vi "AimDetect_VA11_LV2010_R1.vi"(0 "File Path":path=path "c:/$safe$.bmp", 1 "Method (Aim Auto Threshold)":i32(ring)=4 items=["clustering", "entropy", "metric", "moments", "inter-class variance"], 2 "Min Radius (Aim [Blemish/Particle] Detection)":sgl=3.0, 3 "Max Radius (Aim [Blemish/Particle] Detection)":sgl=30.0, 4 "Blemish Percent Contrast":sgl=70.0, 7 "error in":errorcluster) -> (17 "Blemish Threshold Value":sgl=78.026665, 18 "Particle Measurements (Real-World) (AIM [Particle Analysis])":dbl[][](array[numeric]) format="%.2f", 19 "Particle Measurements (Pixels) (AIM [Particle Analysis])":dbl[][](array[numeric])=[[648.3028258887877, 485.8545123062899, 643.0, 443.0, 607.0, 443.0, 689.0, 529.0, 658.0, 443.0, 645.0, 529.0, 607.0, 688.0, 484.0, 82.0, 86.0, 118.82760622010359, 264.80944748205263, 265.4601939773794, 0.0, 86.97700845625813, 91.71967865851053, 76.14199051954876, 80.9379578326276, 66.20236187051316, 66.20236187051316, 93.62427801841118, 63.568523430885826, 56.54639175257732, 58.351063829787236, 20.71300722898772, 83.56864784638057, 5485.0, 1.0, 5486.0, 5529.0, 1228800.0, 1.0, 97.0, 94.0, 94.21744528780259, 81.40408856307903, 0.4463704427083333, 99.98177178271965, 1.2045873509829292, 1.0, 1.3682401880991135, 0.7777935337492909, 1.0086493830001033, 0.9987200812794278, 3555941.0, 2664912.0, 2307595077.0, 1727689606.0, 1297292692.0, 1498960469825.0, 1121182161328.0, 841059124454.0, 632755673718.0, 2268478.006198724, 19625.655059252516, 2533171.900820419, -1261004.9246985912, 1233856.5000050068, 1535799.3924472332, -1340469.0961027145, 0.07540172979257173, 0.0006523353260363689, 0.08419986557589047, -0.0005659462712186631, 0.0005537619018923757, 0.0006892756106429589, -0.0006016102489088325, 0.1596015953684622, 7.910935877209351e-05, 1.2057458860144924e-05, 1.7499590275040425e-08, -7.402347638502482e-15, -1.290757327076249e-10, -3.1338720899899903e-15]] format="%.2f", 20 "Coordinate System Out (Set Coordinate System 1)":T5={"Reference System"={"Origin"={"X"=528.26874, "Y"=474.15033}, "Angle (deg)"=0.0, "Axis Reference"=0}, "Measurement System"={"Origin"={"X"=648.41626, "Y"=485.91132}, "Angle (deg)"=0.0, "Axis Reference"=0}} {"Measurement System"."Axis Reference" items=["Direct", "Indirect"]; "Measurement System"."Angle (deg)" format="%.2f"; "Measurement System"."Origin"."Y" format="%.2f"; "Measurement System"."Origin"."X" format="%.2f"; "Reference System"."Axis Reference" items=["Direct", "Indirect"]; "Reference System"."Angle (deg)" format="%.2f"; "Reference System"."Origin"."Y" format="%.2f"; "Reference System"."Origin"."X" format="%.2f"}, 21 "ROI Pixel Statistics (Aim Line Profile [strength])":T1={"Min"=98.0, "Max"=122.0, "Mean"=111.46667, "Std Dev"=6.1195498, "Count"=15} {"Min" format="%.2f"; "Std Dev" format="%.2f"; "Mean" format="%.2f"; "Max" format="%.2f"}, 22 "Fitted Circle (Aim [Statistics])":T4={"Center (Pixels)"={"X"=648.57495, "Y"=486.02267}, "Radius (Pixels)"=42.87019716746181, "Center (Real-World)"={"X"=648.57495, "Y"=486.02267}, "Radius (Real-World)"=42.87019716746181, "Roundness (Real-World)"=0.08071478631638666, "Average Strength"=75.97746055597301, "Average SNR (dB)"=27.76507581006103} {"Average SNR (dB)" format="%.2f"; "Average Strength" format="%.2f"; "Roundness (Real-World)" format="%.2f"; "Radius (Real-World)" format="%.2f"; "Center (Real-World)"."Y" format="%.2f"; "Center (Real-World)"."X" format="%.2f"; "Radius (Pixels)" format="%.2f"; "Center (Pixels)"."Y" format="%.2f"; "Center (Pixels)"."X" format="%.2f"}, 23 "Nb Circles (Aim [Blemish/Particle] Detection)":i32, 24 "Circles Data (Aim [Blemish/Particle] Detection)":T3(array[cluster]), 25 "Nb Circles (Aim [Number of Circles Found])":i32=1, 26 "Circles Data (Aim [Number of Circles Found])":T3(array[cluster])=[{"Pos. X"=647, "Pos. Y"=486, "Radius"=39, "Core Area"=6}], 27 "error out":errorcluster)   [LabVIEW 2014]
uses:
  <vilib>/vision/Measure.llb/Edge Options.ctl
  <vilib>/vision/Measure.llb/Edge Polarity.ctl
  <vilib>/vision/NI_Vision_Development_Module.lvlib
panel:
  out "Image Out":T2(plugin-control)
  out "Line Profile (Aim Line Profile [strength])":cluster{"x0":sgl, "dx":sgl, "Pixels Line":sgl[]}={"x0"=0.0, "dx"=1.0, "Pixels Line"=[115.0, 108.0, 107.0, 114.0, 118.0, 117.0, 113.0, 110.0, 98.0, 109.0, 108.0, 102.0, 116.0, 115.0, 122.0]} {"Pixels Line" format="%.2f"; "dx" format="%.2f"; "x0" format="%.2f"}
  out "Line Profile Graph":cluster{"x0":sgl, "dx":sgl, "Pixels Line":sgl[]}(graph)={"x0"=0.0, "dx"=1.0, "Pixels Line"=[115.0, 108.0, 107.0, 114.0, 118.0, 117.0, 113.0, 110.0, 98.0, 109.0, 108.0, 102.0, 116.0, 115.0, 122.0]} caption="Line Profile"
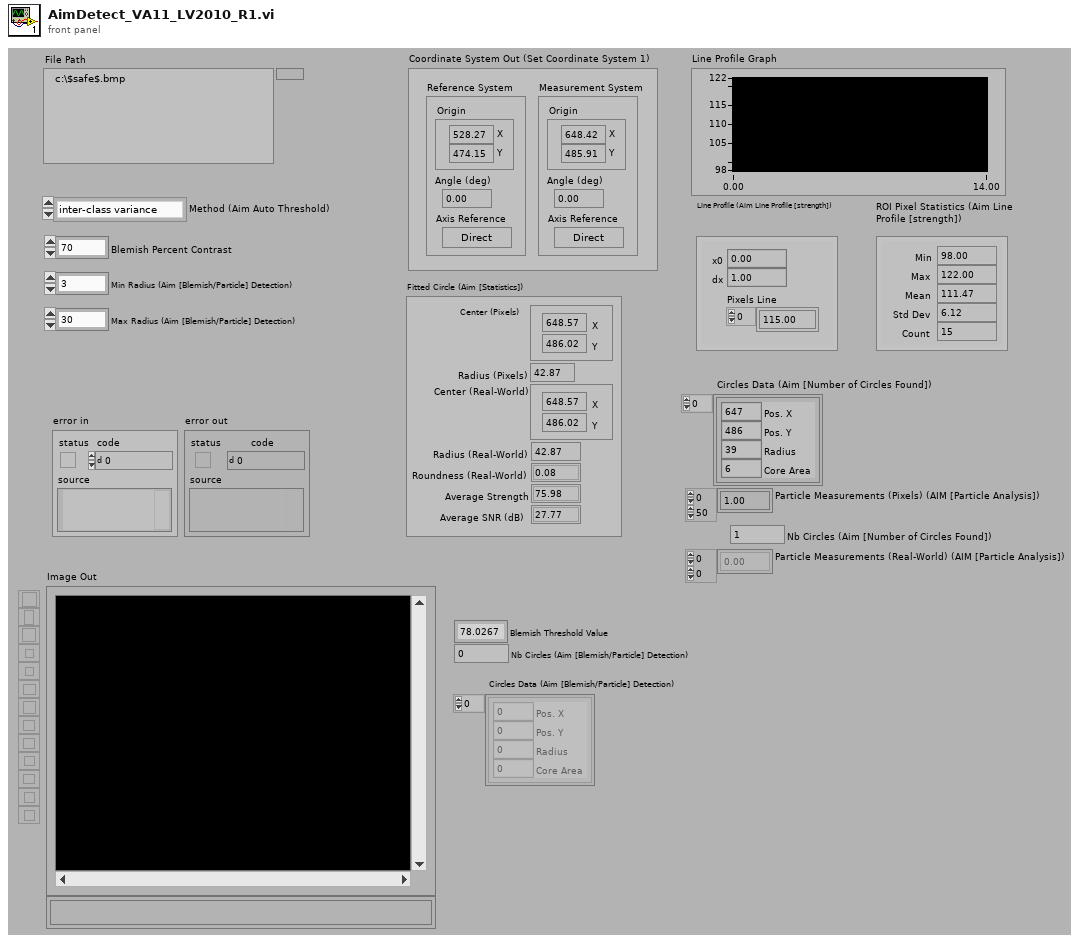
[diagram p1: front panel]
types:
  T1 = cluster{"Min":sgl, "Max":sgl, "Mean":sgl, "Std Dev":sgl, "Count":i32}
  T2 = typedef "IMAQ Image.ctl" = refnum<image>
  T3 = cluster{"Pos. X":i32, "Pos. Y":i32, "Radius":i32, "Core Area":i32}[]
  T4 = cluster{"Center (Pixels)":cluster{"X":sgl, "Y":sgl}, "Radius (Pixels)":dbl, "Center (Real-World)":cluster{"X":sgl, "Y":sgl}, "Radius (Real-World)":dbl, "Roundness (Real-World)":dbl, "Average Strength":dbl, "Average SNR (dB)":dbl}
  T5 = cluster{"Reference System":cluster{"Origin":cluster{"X":sgl, "Y":sgl}, "Angle (deg)":sgl, "Axis Reference":u32}, "Measurement System":cluster{"Origin":cluster{"X":sgl, "Y":sgl}, "Angle (deg)":sgl, "Axis Reference":u32}}
  T6 = cluster{"Global Rectangle":i32[], "Contours":cluster{"ID":enum32{"External", "Internal"}, "Type":u32, "Coordinates":i32[]}[]}
  T7 = typedef "Edge Options.ctl" = cluster{"Edge Polarity":T8, "Kernel Size":u32, "Width":u32, "Minimum Edge Strength":sgl, "Interpolation Type":enum32{"Zero Order", "Bilinear", "Quadratic", "Cubic", "Bilinear Fixed"}, "Data Processing Method":enum32{"Average", "Median"}}
  T8 = typedef "Edge Polarity.ctl" = u32
  T9 = cluster{"Search  Direction":u32, "Edge Options":T7, "Show Search Area":bool, "Show Search Lines":bool, "Show Edges Found":bool, "Show Result":bool, "Search Area Color":u32, "Search Lines Color":u32, "Edge Locations Color":u32, "Result Color":u32, "Overlay Group Name":string}
  T10 = cluster{"Process":enum16{"Get First Edge", "Get First + Last Edge", "Get All Edges", "Get Best Edge"}, "Step Size":i32, "Max Pixel Radius":i32}
  T11 = cluster{"Origin":cluster{"X":sgl, "Y":sgl}, "Angle (deg)":sgl, "Axis Reference":u32}
  T12 = enum16{"Reset", "Update Coordinate System", "Get Coordinate System"}
  T13 = enum16{"Horizontal Motion", "Vertical Motion", "Horizontal and Vertical Motion", "Horizontal, Vertical and Angular Motion"}
  T14 = typedef "Image Type" = u32
  T15 = typedef "IMAQ Coordinate System" = cluster{"Reference System":cluster{"Origin":cluster{"X":sgl, "Y":sgl}, "Angle (deg)":sgl, "Axis Reference":u32}, "Measurement System":cluster{"Origin":cluster{"X":sgl, "Y":sgl}, "Angle (deg)":sgl, "Axis Reference":u32}}
  T16 = typedef "ROI Descriptor" = cluster{"Global Rectangle":i32[], "Contours":cluster{"ID":enum32{"External", "Internal"}, "Type":u32, "Coordinates":i32[]}[]}
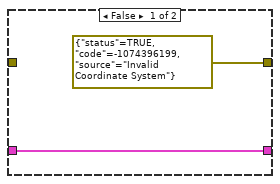
[diagram p4: hidden frame]
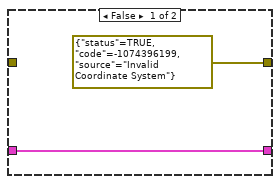
[diagram p6: hidden frame]
diagram:
  (unwired) sgl 0.0 ("y")
  w11 = u32 1 items=["Grayscale", "Binary", "Gradient", "Rainbow", "Temperature", "User Defined"] ("Palette")
  w21 = i32[] [] items=["Center of Mass X", "Center of Mass Y", "First Pixel X", "First Pixel Y", "Bounding Rect Left", "Bounding Rect Top", "Bounding Rect Right", "Bounding Rect Bottom", "Max Feret Diameter Start X", "Max Feret Diameter Start Y", "Max Feret Diameter End X", "Max Feret Diameter End Y", "Max Horiz. Segment Length Left", "Max Horiz. Segment Length Right", "Max Horiz. Segment Length Row", "-", "Bounding Rect Width", "Bounding Rect Height", "Bounding Rect Diagonal", "Perimeter", "Convex Hull Perimeter", "Holes' Perimeter", "Max Feret Diameter", "Equivalent Ellipse Major Axis", "Equivalent Ellipse Minor Axis", "Equivalent Ellipse Minor Axis (Feret)", "Equivalent Rect Long Side", "Equivalent Rect Short Side", "Equivalent Rect Diagonal", "Equivalent Rect Short Side (Feret)", "Average Horiz. Segment Length", "Average Vert. Segment Length", "Hydraulic Radius", "Waddel Disk Diameter", "-", "Area", "Holes' Area", "Particle & Holes' Area", "Convex Hull Area", "Image Area", "-", "Number of Holes", "Number of Horiz. Segments", "Number of Vert. Segments", "-", "Orientation", "Max Feret Diameter Orientation", "-", "% Area/Image Area", "% Area/(Particle & Holes' Area)", "Ratio of Equivalent Ellipse Axes", "Ratio of Equivalent Rect Sides", "-", "Elongation Factor", "Compactness Factor", "Heywood Circularity Factor", "Type Factor", "-", "Sum X", "Sum Y", "Sum XX", "Sum XY", "Sum YY", "Sum XXX", "Sum XXY", "Sum XYY", "Sum YYY", "-", "Moment of Inertia XX", "Moment of Inertia XY", "Moment of Inertia YY", "Moment of Inertia XXX", "Moment of Inertia XXY", "Moment of Inertia XYY", "Moment of Inertia YYY", "Norm. Moment of Inertia XX", "Norm. Moment of Inertia XY", "Norm. Moment of Inertia YY", "Norm. Moment of Inertia XXX", "Norm. Moment of Inertia XXY", "Norm. Moment of Inertia XYY", "Norm. Moment of Inertia YYY", "Hu Moment 1", "Hu Moment 2", "Hu Moment 3", "Hu Moment 4", "Hu Moment 5", "Hu Moment 6", "Hu Moment 7"] ("Real-World Measurements")
  w22 = i32[] [0, 1, 2, 3, 4, 5, 6, 7, 8, 9, 10, 11, 12, 13, 14, 16, 17, 18, 19, 20, 21, 22, 23, 24, 25, 26, 27, 28, 29, 30, 31, 32, 33, 35, 36, 37, 38, 39, 41, 42, 43, 45, 46, 48, 49, 50, 51, 53, 54, 55, 56, 58, 59, 60, 61, 62, 63, 64, 65, 66, 68, 69, 70, 71, 72, 73, 74, 75, 76, 77, 78, 79, 80, 81, 82, 83, 84, 85, 86, 87, 88] items=["Center of Mass X", "Center of Mass Y", "First Pixel X", "First Pixel Y", "Bounding Rect Left", "Bounding Rect Top", "Bounding Rect Right", "Bounding Rect Bottom", "Max Feret Diameter Start X", "Max Feret Diameter Start Y", "Max Feret Diameter End X", "Max Feret Diameter End Y", "Max Horiz. Segment Length Left", "Max Horiz. Segment Length Right", "Max Horiz. Segment Length Row", "-", "Bounding Rect Width", "Bounding Rect Height", "Bounding Rect Diagonal", "Perimeter", "Convex Hull Perimeter", "Holes' Perimeter", "Max Feret Diameter", "Equivalent Ellipse Major Axis", "Equivalent Ellipse Minor Axis", "Equivalent Ellipse Minor Axis (Feret)", "Equivalent Rect Long Side", "Equivalent Rect Short Side", "Equivalent Rect Diagonal", "Equivalent Rect Short Side (Feret)", "Average Horiz. Segment Length", "Average Vert. Segment Length", "Hydraulic Radius", "Waddel Disk Diameter", "-", "Area", "Holes' Area", "Particle & Holes' Area", "Convex Hull Area", "Image Area", "-", "Number of Holes", "Number of Horiz. Segments", "Number of Vert. Segments", "-", "Orientation", "Max Feret Diameter Orientation", "-", "% Area/Image Area", "% Area/(Particle & Holes' Area)", "Ratio of Equivalent Ellipse Axes", "Ratio of Equivalent Rect Sides", "-", "Elongation Factor", "Compactness Factor", "Heywood Circularity Factor", "Type Factor", "-", "Sum X", "Sum Y", "Sum XX", "Sum XY", "Sum YY", "Sum XXX", "Sum XXY", "Sum XYY", "Sum YYY", "-", "Moment of Inertia XX", "Moment of Inertia XY", "Moment of Inertia YY", "Moment of Inertia XXX", "Moment of Inertia XXY", "Moment of Inertia XYY", "Moment of Inertia YYY", "Norm. Moment of Inertia XX", "Norm. Moment of Inertia XY", "Norm. Moment of Inertia YY", "Norm. Moment of Inertia XXX", "Norm. Moment of Inertia XXY", "Norm. Moment of Inertia XYY", "Norm. Moment of Inertia YYY", "Hu Moment 1", "Hu Moment 2", "Hu Moment 3", "Hu Moment 4", "Hu Moment 5", "Hu Moment 6", "Hu Moment 7"] ("Pixel Measurements")
  w17 = TRUE ("Connectivity 4/8 (8)")
  w65 = T6 {"Global Rectangle"=[391, 135, 821, 527], "Contours"=[{"ID"=enum."External", "Type"=4, "Coordinates"=[380, 194, 990, 772]}]}  # ROI Descriptor
  w106 = u16 1 items=["Push", "Pop", "Reset"] ("Function")
  w111 = T6 {"Global Rectangle"=[140, 84, 1113, 700], "Contours"=[{"ID"=enum."External", "Type"=3, "Coordinates"=[140, 84, 1113, 700]}]}  # ROI Descriptor
  w115 = u32 0 items=["Bright Objects", "Dark Objects"] ("Look For")
  w120 = u16 0 items=["Push", "Pop", "Reset"] ("Function")
  w123 = u32 0 items=["Horizontal", "Vertical", "Central", "1st Diagonal", "2nd Diagonal"] ("Type of Symmetry")
  w126 = T14 0 items=["Grayscale (U8)", "Grayscale (I16)", "Grayscale (SGL)", "Complex (CSG)", "RGB (U32)", "HSL (U32)", "RGB (U64)", "Grayscale (U16)"] ("Image Type")
  # "Reverse the image."
  # "Reverse the image."
  # "Buffer"
  # "Buffer"
  n1 = Call Chain() -> (call chain=w128:string[])
  n2 = Index Array(array=w128) -> (element=w127:string)  [unwired: 1 in]
  n3 = call "IMAQ Create"("Image Name"=w127, "Image Type"=w126, "error in (no error)"="error in") -> ("New Image"=w131:T2, "error out"=w130:errorcluster)  [unwired: 1 in, 1 out]
  n4 = call "IMAQ ReadFile"("File Path"="File Path", "error in (no error)"=w130, "Image"=w131) -> ("error out"=w132:errorcluster, "Image Out"=w125:T2)  [unwired: 2 in, 5 out]
  n5 = call "IMAQ Symmetry"("error in (no error)"=w132, "Type of Symmetry"=w123, "Image Src"=w125) -> ("error out"=w124:errorcluster, "Image Dst Out"=w122:T2)  [unwired: 1 in, 1 out]
  n6 = call <vilib>:"IVA Image Buffer.vi"("Function"=w120, "error in (no error)"=w124, "Prefix"="vision assistant", "Buffer #"=0, "Image In"=w122) -> ("error out"=w121:errorcluster, "Image Out"=w117:T2)  [unwired: 5 out]
  n7 = call "IMAQ AutoBThreshold 2"("Image Src"=w117, "Look For (Bright Objects)"=w115, "Method (clustering)"="Method (Aim Auto Threshold)", "error in (no error)"=w121) -> ("Image Dst Out"=w112:T2, "error out"=w116:errorcluster)  [unwired: 4 in, 6 out]
  n8 = Unbundle By Name(w116) -> ("code"=w109:i32)
  n9 = case shown="Default" w109 {
    tunnel: w116 -> [_ w144]
    tunnel: [_ w143] -> w113
    tunnel: w112 -> [w133 w141]
    tunnel: [w133 w140] -> w108
    tunnel: [_ w139] -> _
    tunnel: [_ w138] -> _
    tunnel: w111 -> [_ w137]
    tunnel: "Aim Centroid" ("Step Name") -> [_ w134]
    frame -1074396199, -1074396198 {
      # "Discard Coordinate System Error"
    }
    frame Default {
      # "Create an image mask to apply the centroid\non a specific region of the image."
      n10 = call "IMAQ Create"("Image Name"="Image Mask", "error in (no error)"=w144) -> ("New Image"=w147:T2, "error out"=w146:errorcluster)  [unwired: 2 in, 1 out]
      n11 = call "IMAQ ROIToMask"("error in (no error)"=w146, "ROI Descriptor"=w137, "Image"=w147) -> ("error out"=w142:errorcluster, "Image Out"=w145:T2)  [unwired: 2 in, 2 out]
      n12 = call "IMAQ Centroid"("error in (no error)"=w142, "Image Mask"=w145, "Image"=w141) -> ("error out"=w136:errorcluster, "Centroid"=w139:cluster{"X Centroid":sgl, "Y Centroid":sgl})  [unwired: 1 out]
      n13 = call <vilib>:"IVA Store Centroid Results.vi"("Centroid in"=w139, "error in (no error)"=w136, "Step Name"=w134, "Image in"=w141) -> ("error out"=w135:errorcluster, "Image dup"=w140:T2, "Calibrated Centroid"=w138:cluster{"X":sgl, "Y":sgl})  [unwired: 5 out]
      n14 = call "Imaq Dispose"("Image"=w147, "error in (no error)"=w135) -> ("error out"=w143:errorcluster)  [unwired: 1 in, 3 out]
    }
  }
  n15 = call <vilib>:"IVA Image Buffer.vi"("Function"=w106, "error in (no error)"=w113, "Prefix"="vision assistant", "Buffer #"=0, "Image In"=w108) -> ("error out"=w107:errorcluster, "Image Out"=w84:T2)  [unwired: 5 out]
  n16 = call <vilib>:"IVA Coordinate System Manager 2.vi"("Mode"=T13."Horizontal and Vertical Motion", "Reference System"=T11 {"Origin"={"X"=528.26874, "Y"=474.15033}, "Angle (deg)"=0.0, "Axis Reference"=0}, "Function"=T12."Update Coordinate System", "error in (no error)"=w107, "Angle ID"=cluster{"GUID":string, "Index":i32} {"GUID"="", "Index"=0}, "Origin ID"=cluster{"GUID":string, "Index":i32} {"GUID"="Aim Centroid", "Index"=0}, "Coordinate System Name"="Set Coordinate System 1") -> ("error out"=w97:errorcluster, "Coordinate System Out"=→"Coordinate System Out (Set Coordinate System 1)":T15)  [unwired: 3 out]
  n17 = call <vilib>:"IVA Coordinate System Manager 2.vi"("Reference System"=T11 {"Origin"={"X"=605.7612, "Y"=332.0605}, "Angle (deg)"=0.0, "Axis Reference"=0}, "Function"=T12."Get Coordinate System", "error in (no error)"=w97, "Coordinate System Name"="Set Coordinate System 1") -> ("error out"=w93:errorcluster, "Coordinate System Out"=w89:T15)  [unwired: 3 in, 3 out]
  n18 = call <vilib>:"IVA Check Coordinate System Valid.vi"("Coordinate System"=w89) -> ("Valid?"=w88:bool)
  n19 = case shown="True" w88 {
    tunnel: T6 {"Global Rectangle"=[601, 325, 611, 340], "Contours"=[{"ID"=enum."External", "Type"=2, "Coordinates"=[601, 325, 610, 339]}]} ("ROI Descriptor") -> [w149 w157]
    tunnel: [w149 w154] -> w83
    tunnel: [errorcluster {"status"=TRUE, "code"=-1074396199, "source"="Invalid Coordinate System"} ("error out") w153] -> w90
    tunnel: w89 -> [_ w152]
    tunnel: w93 -> [_ w151]
    frame False {
    }
    frame True {
      n20 = Unbundle By Name(w152) -> ("Reference System"=w156:T11, "Measurement System"=w155:T11)
      n21 = call "IMAQ TransformROI"("error in (no error)"=w151, "New Reference"=w155, "Base Reference"=w156, "ROI Descriptor"=w157) -> ("error out"=w153:errorcluster, "ROI Descriptor out"=w154:T16)  [unwired: 6 out]
    }
  }
  n22 = Unbundle By Name(w90) -> ("code"=w82:i32)
  n23 = case shown="Default" w82 {
    tunnel: w90 -> [_ w164]
    tunnel: [_ w163] -> w7
    tunnel: [_ w162] -> w86
    tunnel: w84 -> [w158 w159]
    tunnel: [_ w161] -> w8
    tunnel: w83 -> [_ w160]
    tunnel: [w158 w159] -> w73
    frame -1074396199, -1074396198 {
      # "Discard\nCoordinate\nSystem\nError"
    }
    frame Default {
      n24 = call "IMAQ ROIProfile"("error in (no error)"=w164, "ROI Descriptor"=w160, "Image"=w159) -> ("ROI Pixel Statistics"=w163:T1, "error out"=w162:errorcluster, "ROI Graph"=w161:cluster{"x0":sgl, "dx":sgl, "Pixels Line":sgl[]})  [unwired: 3 out]
    }
  }
  "Line Profile Graph" <- w8
  "Line Profile (Aim Line Profile [strength])" <- w8
  "ROI Pixel Statistics (Aim Line Profile [strength])" <- w7
  n25 = property on="Line Profile Graph" class="WFGraph (strict)"(error in=w86, "Y Scale.Mapping Mode"=u8 0) -> (error out=w85:errorcluster)  [unwired: 1 in, 1 out]
  n26 = call <vilib>:"IVA Coordinate System Manager 2.vi"("Reference System"=T11 {"Origin"={"X"=605.7612, "Y"=332.0605}, "Angle (deg)"=0.0, "Axis Reference"=0}, "Function"=T12."Get Coordinate System", "error in (no error)"=w85, "Coordinate System Name"="Set Coordinate System 1") -> ("error out"=w79:errorcluster, "Coordinate System Out"=w75:T15)  [unwired: 3 in, 3 out]
  n27 = call <vilib>:"IVA Check Coordinate System Valid.vi"("Coordinate System"=w75) -> ("Valid?"=w74:bool)
  n28 = case shown="True" w74 {
    tunnel: T6 {"Global Rectangle"=[352, 79, 856, 582], "Contours"=[{"ID"=enum."External", "Type"=7, "Coordinates"=[603, 330, 7, 251, 0, 0]}]} ("ROI Descriptor") -> [w165 w173]
    tunnel: [w165 w170] -> w70
    tunnel: [errorcluster {"status"=TRUE, "code"=-1074396199, "source"="Invalid Coordinate System"} ("error out") w169] -> w76
    tunnel: w75 -> [_ w168]
    tunnel: w79 -> [_ w167]
    frame False {
    }
    frame True {
      n29 = Unbundle By Name(w168) -> ("Reference System"=w172:T11, "Measurement System"=w171:T11)
      n30 = call "IMAQ TransformROI"("error in (no error)"=w167, "New Reference"=w171, "Base Reference"=w172, "ROI Descriptor"=w173) -> ("error out"=w169:errorcluster, "ROI Descriptor out"=w170:T16)  [unwired: 6 out]
    }
  }
  n31 = Unbundle By Name(w76) -> ("code"=w69:i32)
  n32 = case shown="Default" w69 {
    tunnel: T9 {"Search  Direction"=1, "Edge Options"={"Edge Polarity"=2, "Kernel Size"=13, "Width"=13, "Minimum Edge Strength"=35.0, "Interpolation Type"=enum."Bilinear Fixed", "Data Processing Method"=enum."Average"}, "Show Search Area"=TRUE, "Show Search Lines"=TRUE, "Show Edges Found"=TRUE, "Show Result"=TRUE, "Search Area Color"=65280, "Search Lines Color"=255, "Edge Locations Color"=16776960, "Result Color"=16711680, "Overlay Group Name"=""} ("Options") -> [_ w175]
    tunnel: w73 -> [w174 w185]
    tunnel: w76 -> [_ w184]
    tunnel: [_ w182] -> w72
    tunnel: [w174 w180] -> w63
    tunnel: "Aim [Statistics]" ("Step Name") -> [_ w179]
    tunnel: w70 -> [_ w178]
    tunnel: T10 {"Process"=enum."Get First Edge", "Step Size"=3, "Max Pixel Radius"=3} ("Circle Fit Options") -> [_ w177]
    tunnel: [_ w176] -> w67
    frame -1074396199, -1074396198 {
      # "Discard Coordinate System Error"
    }
    frame Default {
      n33 = call "IMAQ Find Circular Edge 2"("Circle Fit Options"=w177, "Options"=w175, "error in (no error)"=w184, "ROI Descriptor"=w178, "Image"=w185) -> ("error out"=w183:errorcluster, "Fitted Circle"=w176:T4, "Image Out"=w181:T2)  [unwired: 1 in, 3 out]
      n34 = call <vilib>:"IVA Store Circular Edge2 Results.vi"("error in (no error)"=w183, "Step Name"=w179, "Fitted Circle"=w176, "Image in"=w181) -> ("error out"=w182:errorcluster, "Image dup"=w180:T2)  [unwired: 2 in, 4 out]
    }
  }
  "Fitted Circle (Aim [Statistics])" <- w67
  n35 = Unbundle By Name(w72) -> ("code"=w60:i32)
  n36 = case "IVA Mask from ROI" shown="Default" w60 {
    tunnel: w65 -> [_ w193]
    tunnel: FALSE ("Shrink") -> [_ w192]
    tunnel: w63 -> [w186 w191]
    tunnel: w72 -> [_ w190]
    tunnel: [_ w189] -> w62
    tunnel: [w186 w188] -> w58
    tunnel: FALSE ("Out / In") -> [_ w187]
    frame -1074396199, -1074396198 {
      # "Discard\nCoordinate\nSystem\nError"
    }
    frame Default {
      n37 = call <vilib>:"IVA Mask from ROI.vi"("Shrink"=w192, "ROI Descriptor"=w193, "error in (no error)"=w190, "Out / In"=w187, "Image Src"=w191) -> ("error out"=w189:errorcluster, "Image Out"=w188:T2)  [unwired: 5 out]
    }
  }
  n38 = Unbundle By Name(w7) -> ("Mean"=w4:sgl)
  n39 = Divide(x="Blemish Percent Contrast", y=sgl 100.0) -> (x/y=w3:sgl)
  n40 = Multiply(x=w3, y=w4) -> (x*y=w5:sgl)
  "Blemish Threshold Value" <- w5
  n41 = Bundle By Name(cluster=cluster{"Lower value":sgl, "Upper value":sgl} {"Lower value"=81.0, "Upper value"=255.0} ("Range (Aim Quality [Manual Threshold])"), "Lower value"=w5) -> (w6:cluster{"Lower value":sgl, "Upper value":sgl})
  n42 = call "IMAQ Threshold"("error in (no error)"=w62, "Range"=w6, "Image Src"=w58) -> ("error out"=w57:errorcluster, "Image Dst Out"=w56:T2)  [unwired: 3 in, 4 out]
  n43 = call <vilib>:"IVA Binary Inverse.vi"("error in (no error)"=w57, "Image In"=w56) -> ("error out"=w55:errorcluster, "Image Out"=w45:T2)  [unwired: 8 out]
  n44 = call "IMAQ Create"("Image Name"="Circle Image", "error in (no error)"=w55) -> ("New Image"=w50:T2, "error out"=w49:errorcluster)  [unwired: 2 in, 1 out]
  n45 = call "IMAQ Find Circles"("Max Radius"="Max Radius (Aim [Blemish/Particle] Detection)", "error in (no error)"=w49, "Min Radius"="Min Radius (Aim [Blemish/Particle] Detection)", "Image Dst"=w50, "Image Src"=w45) -> ("error out"=w48:errorcluster, "Circles Data"=w43:T3, "Nb Circles"=→"Nb Circles (Aim [Blemish/Particle] Detection)":i32)  [unwired: 4 out]
  "Circles Data (Aim [Blemish/Particle] Detection)" <- w43
  n46 = call "Imaq Dispose"("Image"=w50, "error in (no error)"=w48) -> ("error out"=w47:errorcluster)  [unwired: 1 in, 3 out]
  n47 = call <vilib>:"IVA Store Circles Results.vi"("error in (no error)"=w47, "Circles Data"=w43, "Step Name"="Aiim [Blemish/Particle] Detection", "Image in"=w45) -> ("error out"=w46:errorcluster, "Image dup"=w42:T2)  [unwired: 6 out]
  n48 = call <vilib>:"IVA Binary Inverse.vi"("error in (no error)"=w46, "Image In"=w42) -> ("error out"=w41:errorcluster, "Image Out"=w36:T2)  [unwired: 8 out]
  n49 = call "IMAQ RemoveParticle"("Connectivity 4/8 (8)"=TRUE, "Low Pass/High Pass (Low)"=FALSE, "Square/Hexa (Square)"=FALSE, "error in (no error)"=w41, "Number of Erosion"=1, "Image Src"=w36) -> ("error out"=w35:errorcluster, "Image Dst Out"=w25:T2)  [unwired: 1 in, 3 out]
  n50 = call "IMAQ Create"("Image Name"="Circle Image", "error in (no error)"=w35) -> ("New Image"=w30:T2, "error out"=w29:errorcluster)  [unwired: 2 in, 1 out]
  n51 = call "IMAQ Find Circles"("Max Radius"=sgl 300.0 ("Max Radius (Aim [Number of Circles Found])"), "error in (no error)"=w29, "Min Radius"=sgl 3.0 ("Min Radius (Aim [Number of Circles Found])"), "Image Dst"=w30, "Image Src"=w25) -> ("error out"=w28:errorcluster, "Circles Data"=w23:T3, "Nb Circles"=→"Nb Circles (Aim [Number of Circles Found])":i32)  [unwired: 4 out]
  "Circles Data (Aim [Number of Circles Found])" <- w23
  n52 = call "Imaq Dispose"("Image"=w30, "error in (no error)"=w28) -> ("error out"=w27:errorcluster)  [unwired: 1 in, 3 out]
  n53 = call <vilib>:"IVA Store Circles Results.vi"("error in (no error)"=w27, "Circles Data"=w23, "Step Name"="Aim [Number of Circles Found]", "Image in"=w25) -> ("error out"=w26:errorcluster, "Image dup"=w18:T2)  [unwired: 6 out]
  n54 = call "IMAQ Particle Analysis"("Connectivity 4/8 (8)"=w17, "error in (no error)"=w26, "Real-World Measurements"=w21, "Pixel Measurements"=w22, "Image"=w18) -> ("error out"=w14:errorcluster, "Particle Measurements (Real-World)"=→"Particle Measurements (Real-World) (AIM [Particle Analysis])":dbl[][], "Particle Measurements (Pixels)"=→"Particle Measurements (Pixels) (AIM [Particle Analysis])":dbl[][], "Image Out (duplicate)"=w16:T2)  [unwired: 3 out]
  n55 = call <vilib>:"IVA Store Particles Results.vi"("error in (no error)"=w14, "Connectivity 4/8 (8)"=w17, "Step Name"="AIM [Particle Analysis]", "Image in"=w16) -> ("error out"=w13:errorcluster, "Image dup"=→"Image Out":T2)  [unwired: 6 out]
  n56 = property on="Image Out" class="ImageControl"(error in=w13, "Palette:Palette Type"=w11) -> (error out=→"error out":errorcluster)  [unwired: 1 in, 1 out]
